vi "test-main.vi"() -> ()   [LabVIEW 2013]
uses:
  <vilib>/picture/3D Picture Control/NI_3D Picture Control.lvlib
panel:
  out "Angle":sgl caption="角"
  out "Axis":cluster{"X":sgl, "Y":sgl, "Z":sgl} caption="轴"
  in  "Angle 8":i32(slide) scale=-45.0..180.0
  in  "Angle 7":i32(slide) scale=-45.0..180.0
  in  "停止按钮":bool
  in  "Angle 6":i32(slide) scale=-45.0..180.0
  out "Display":refnum<vi>(3d-picture)
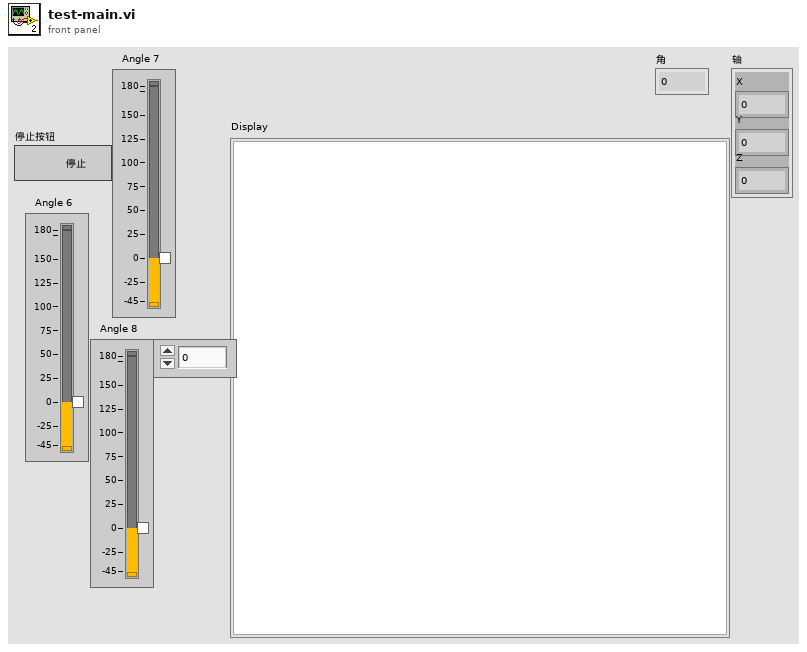
[diagram p1: front panel]
types:
  T1 = cluster{"zuoqian1":refnum<vi>, "zuoqian2":refnum<vi>, "zuoqian3":refnum<vi>}
  T2 = cluster{"zuohou1":refnum<vi>, "zuohou2":refnum<vi>, "zuohou3":refnum<vi>}
  T3 = cluster{"youqian1":refnum<vi>, "youqian2":refnum<vi>, "youqian3":refnum<vi>}
  T4 = cluster{"youhou1":refnum<vi>, "youhou2":refnum<vi>, "youhou3":refnum<vi>}
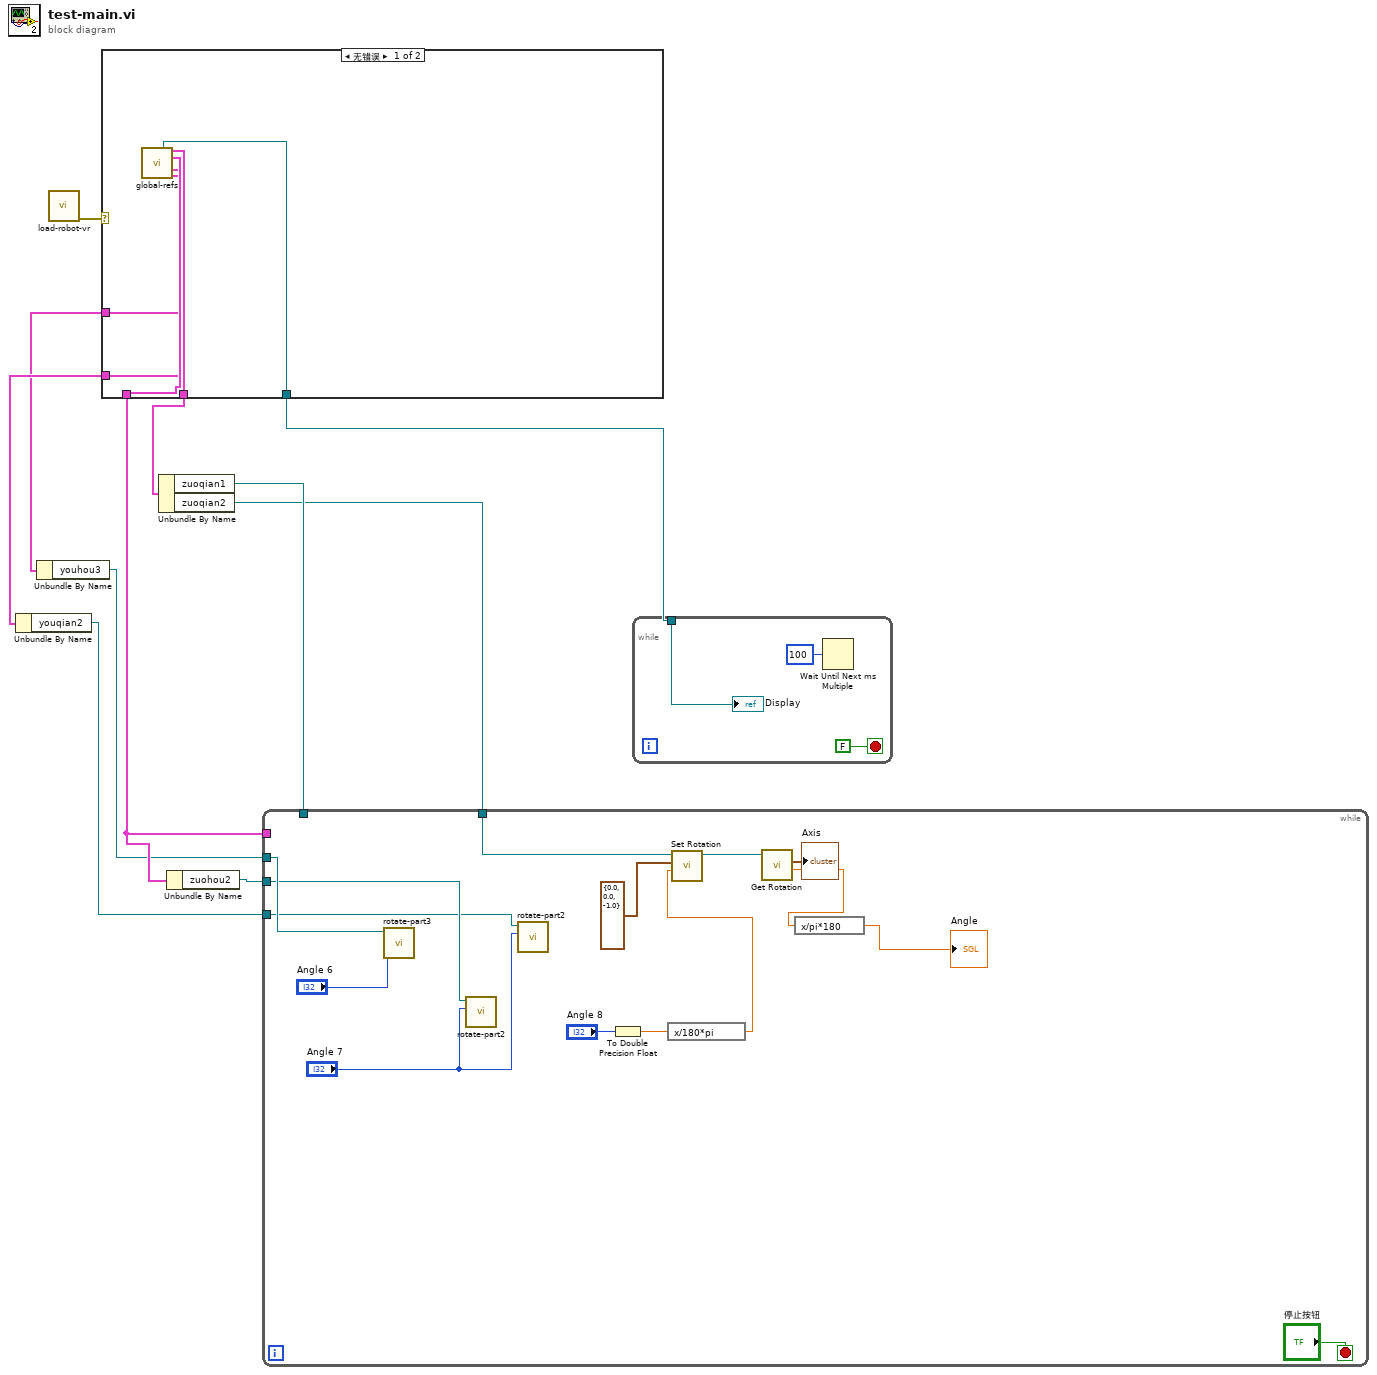
[diagram p0: block diagram]
diagram:
  n1 = call "load-robot-vr.vi"() -> ("错误输出"=w11:errorcluster)  [unwired: 11 in]
  n2 = case shown="无错误" w11 {
    tunnel: [w16 _] -> w2
    tunnel: [w15 _] -> w10
    tunnel: [w14 _] -> w9
    tunnel: [w13 _] -> w6
    tunnel: [w12 _] -> w4
    frame No Error {
      n3 = call "global-refs.vi"() -> ("RobotRef"=w16:refnum<vi>, "ZuoQianRef"=w15:T1, "ZuoHouRef"=w14:T2, "YouQianRef"=w13:T3, "YouHouRef"=w12:T4)  [unwired: 10 in, 1 out]
    }
    frame Error {
    }
  }
  n4 = Unbundle By Name(w6) -> ("youqian2"=w5:refnum<vi>)
  n5 = Unbundle By Name(w4) -> ("youhou3"=w3:refnum<vi>)
  n6 = Unbundle By Name(w10) -> ("zuoqian1"=w7:refnum<vi>, "zuoqian2"=w1:refnum<vi>)
  n7 = Unbundle By Name(w9) -> ("zuohou2"=w8:refnum<vi>)
  n8 = while {
    tunnel: w9 -> [_]
    tunnel: w8 -> [w28]
    tunnel: w7 -> [_]
    tunnel: w5 -> [w27]
    tunnel: w3 -> [w29]
    tunnel: w1 -> [w25]
    stop <- "停止按钮" stop-if-true
    n9 = call "rotate-part3.vi"("Angle"="Angle 6", "SceneObject输入"=w29) -> ()  [unwired: 10 in]
    n10 = call "rotate-part2.vi"("Angle"="Angle 7", "SceneObject输入"=w28) -> ()  [unwired: 10 in]
    n11 = call "rotate-part2.vi"("Angle"="Angle 7", "SceneObject输入"=w27) -> ()  [unwired: 10 in]
    n12 = To Double Precision Float(number="Angle 8") -> (double precision float=w23:dbl)
    n13 = expression code="x/180*pi"(w23) -> (w21:dbl)
    n14 = call <vilib>:"Set Rotation.vi"("Angle"=w21, "Axis"=cluster{"X":sgl, "Y":sgl, "Z":sgl} {"X"=0.0, "Y"=0.0, "Z"=-1.0}, "Scene Object"=w25) -> ("Rotated Scene Object"=w20:refnum<vi>)  [unwired: 7 in, 1 out]
    n15 = call <vilib>:"Get Rotation.vi"("Scene Object"=w20) -> ("Angle"=w18:sgl, "Axis"=→"Axis":cluster{"X":sgl, "Y":sgl, "Z":sgl})  [unwired: 7 in, 2 out]
    n16 = expression code="x/pi*180"(w18) -> (→"Angle":sgl)
  }
  n17 = while {
    tunnel: w2 -> [w34]
    stop <- FALSE stop-if-true
    n18 = Wait Until Next ms Multiple(millisecond multiple=u32 100 ("毫秒倍数")) -> ()  [unwired: 1 out]
    "Display" <- w34
  }
